vi "Lockin.LocalClient.vi"(8 "error in (no error)":errorcluster, 9 "Data":variant, 10 "Command":variant, 11 "Instrument.Lockin in":refnum<class "Instrument.Lockin.lvclass">) -> (0 "error out":errorcluster, 3 "Instrument.Lockin out":refnum<class "Instrument.Lockin.lvclass">)   [LabVIEW 2019, in "Instrument.Lockin.lvclass"]
uses:
  Instrument.Lockin.lvclass
  ab83c8ec-e79e-45f6-bac9-d64b8ff87d9e.vi
  3ff62c5d-2582-4752-b0f3-831d8d209e05.vi
  <userlib>/LevyLab/Instrument Framework/Instrument/Instrument.lvclass
  <userlib>/LevyLab/Instrument Framework/Instrument/API/Instrument.sendMessageToProcess (string).vi
  C:/Program Files (x86)/National Instruments/LabVIEW 2019/user.lib/LevyLab/Instrument Framework/Instrument Types/Lockin/Instrument.LockinAPI.lvclass
  C:/Program Files (x86)/National Instruments/LabVIEW 2019/user.lib/LevyLab/Instrument Framework/Instrument/Instrument.lvclass
  C:/Program Files (x86)/National Instruments/LabVIEW 2019/vi.lib/JKI/JKI SMO/SMO/SMO.lvclass
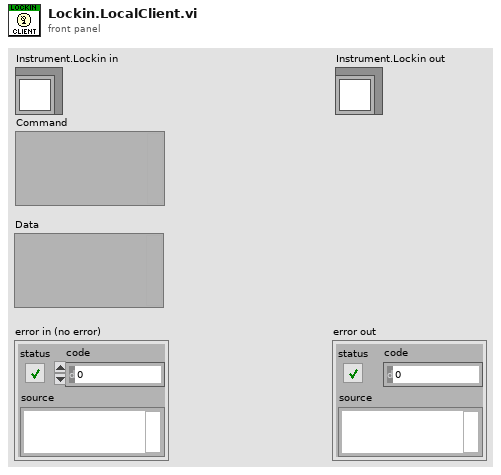
[diagram p1: front panel]
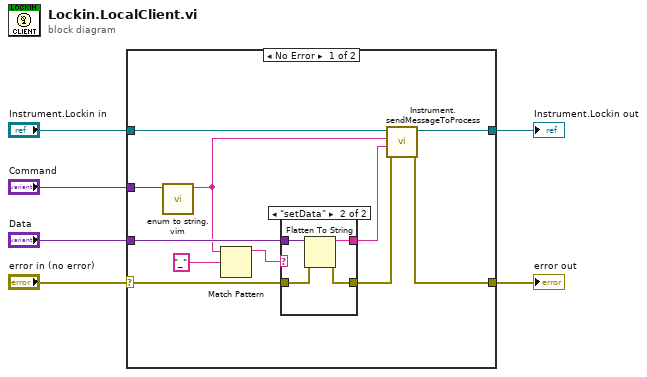
[diagram p0: block diagram]
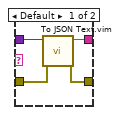
[diagram p2: hidden frame]
diagram:
  n1 = case shown="No Error" "error in (no error)" {
    selector: "error in (no error)" -> [w11 w27]
    tunnel: "Data" -> [w13 _]
    tunnel: [w14 w27] -> w5
    tunnel: "Command" -> [w15 _]
    tunnel: "Instrument.Lockin in" -> [w17 w26]
    tunnel: [w16 w26] -> w1
    frame No Error {
      n2 = call "enum to string.vim"("enum in"=w15) -> ("string out"=w7:string)  [unwired: 9 in, 1 out]
      n3 = Match Pattern(string=w7, regular expression="_") -> (before substring=w8:string)  [unwired: 1 in, 3 out]
      n4 = case shown="\"setData\"" w8 {
        tunnel: w13 -> [w21 w25]
        tunnel: [w20 w24] -> w12
        tunnel: w11 -> [w19 w23]
        tunnel: [w18 w22] -> w10
        frame Default {
          n5 = call "To JSON Text.vim"("error in (no error)"=w19, "Anything"=w21) -> ("error out"=w18:errorcluster, "<JSON>"=w20:string)  [unwired: 8 in]
        }
        frame "setData" {
          n6 = Flatten To String(anything=w25, error in (no error)=w23) -> (data string=w24:string, error out=w22:errorcluster)  [unwired: 2 in, 1 out]
        }
      }
      n7 = call-poly <userlib>:"Instrument.sendMessageToProcess.vi"("error in (no error)"=w10, "Data"=w12, "Command"=w7, "Instrument"=w17) -> ("error out"=w14:errorcluster, "Instrument out"=w16:refnum<class "Instrument.Lockin.lvclass">)  [unwired: 6 in]
    }
    frame Error {
    }
  }
  "Instrument.Lockin out" <- w1
  "error out" <- w5
